vi "Write equinoxPrefix.vi"(8 "error in (no error)":errorcluster, 10 "equinoxPrefix":T1, 11 "RADecParameters in":refnum<class "RADecParameters.lvclass">) -> (0 "error out":errorcluster, 3 "RADecParameters out":refnum<class "RADecParameters.lvclass">)   [LabVIEW 2022 SP3, in "TCSDataDefinitions.lvlib" / "TCSCommand.lvlib" / "TargetConfiguration.lvlib" / "Target.lvlib" / "FixedTarget.lvlib" / "RADecParameters.lvclass"]
uses:
  RADecParameters.lvclass
  Enumerations/EquinoxPrefix.ctl
  RADecParameters.lvclass/RADecParameters.ctl
  FixedTarget.lvlib
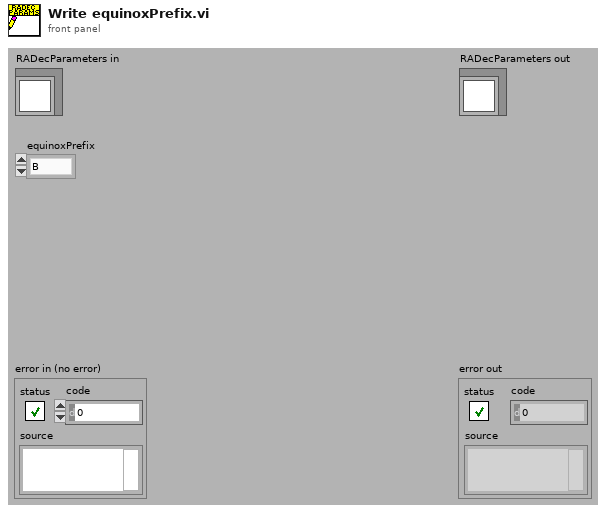
[diagram p1: front panel]
types:
  T1 = typedef "TCSDataDefinitions.lvlib/TCSCommand.lvlib/TargetConfiguration.lvlib/Target.lvlib/FixedTarget.lvlib/EquinoxPrefix.ctl" = enum16{"B", "J"}
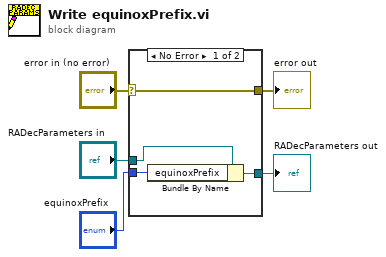
[diagram p0: block diagram]
diagram:
  n1 = case shown="No Error" "error in (no error)" {
    selector: "error in (no error)" -> [w9 w10]
    tunnel: [w9 w10] -> w4
    tunnel: [w7 w11] -> w2
    tunnel: "RADecParameters in" -> [w8 w11]
    tunnel: "equinoxPrefix" -> [w6 _]
    frame No Error {
      n2 = Bundle By Name(cluster=w8, "equinoxPrefix"=w6) -> (w7:refnum<class "RADecParameters.lvclass">)
    }
    frame Error {
    }
  }
  "error out" <- w4
  "RADecParameters out" <- w2
